vi "Mouse Move (Deprecated).vi"(7 "Map Model in":refnum<class "Map Model.lvclass">, 8 "error in (no error)":errorcluster, 10 "Position":T1, 11 "Eraser in":refnum<class "Eraser.lvclass">) -> (0 "error out":errorcluster, 3 "Eraser out":refnum<class "Eraser.lvclass">, 5 "Map Model out":refnum<class "Map Model.lvclass">)   [LabVIEW 2020, in "Map Model.lvlib" / "Eraser.lvclass"]
uses:
  Eraser.lvclass
  <vilib>/Utility/miscctls.llb/LVPoint32TypeDef.ctl
  Map Model/Map Model.lvclass
  Tool/Tool.lvclass
  Undoable Tool/Undoable Tool.lvclass
  E:/Project/Labview-Projects/Completed projects/Map Editor/Models/Map Model/Tools/Undoable Tool/Undoable Tool.lvclass
  E:/Project/Labview-Projects/Completed projects/Map Editor/Models/Map Model/Tools/Tool/Tool.lvclass
panel:
  # "NOTICE -- YOU MUST LEAVE THIS NOTICE IN PLACE.\n\nCopyright (c) 2017, LIANG LIU Shawn.Liu.cn@gmail.com\nAll rights reserved.\n\nRedistribution and use in source and binary forms, with or without modification, are permitted provided that the following conditions are met:\n-Redistributions of source code must retain the above copyright notice, this list of conditions and the following disclaimer.\n-Redistributions in binary form must reproduce the above copyright notice, this list of conditions and the following disclaimer in the documentation and/or other materials provided with the distribution.\n-Neither the name of the eLp nor the names of its contributors may be used to endorse or promote products derived from this software without specific prior written permission.\n\nTHIS SOFTWARE IS PROVIDED BY THE COPYRIGHT HOLDERS AND CONTRIBUTORS \"AS IS\" AND ANY EXPRESS OR IMPLIED WARRANTIES, INCLUDING, BUT NOT LIMITED TO, THE IMPLIED WARRANTIES OF MERCHANTABILITY AND FITNESS FOR A PARTICULAR PURPOSE ARE DISCLAIMED. IN NO EVENT SHALL THE COPYRIGHT HOLDER OR CONTRIBUTORS BE LIABLE FOR ANY DIRECT, INDIRECT, INCIDENTAL, SPECIAL, EXEMPLARY, OR CONSEQUENTIAL DAMAGES (INCLUDING, BUT NOT LIMITED TO, PROCUREMENT OF SUBSTITUTE GOODS OR SERVICES; LOSS OF USE, DATA, OR PROFITS; OR BUSINESS INTERRUPTION) HOWEVER CAUSED AND ON ANY THEORY OF LIABILITY, WHETHER IN CONTRACT, STRICT LIABILITY, OR TORT (INCLUDING NEGLIGENCE OR OTHERWISE) ARISING IN ANY WAY OUT OF THE USE OF THIS SOFTWARE, EVEN IF ADVISED OF THE POSSIBILITY OF SUCH DAMAGE."
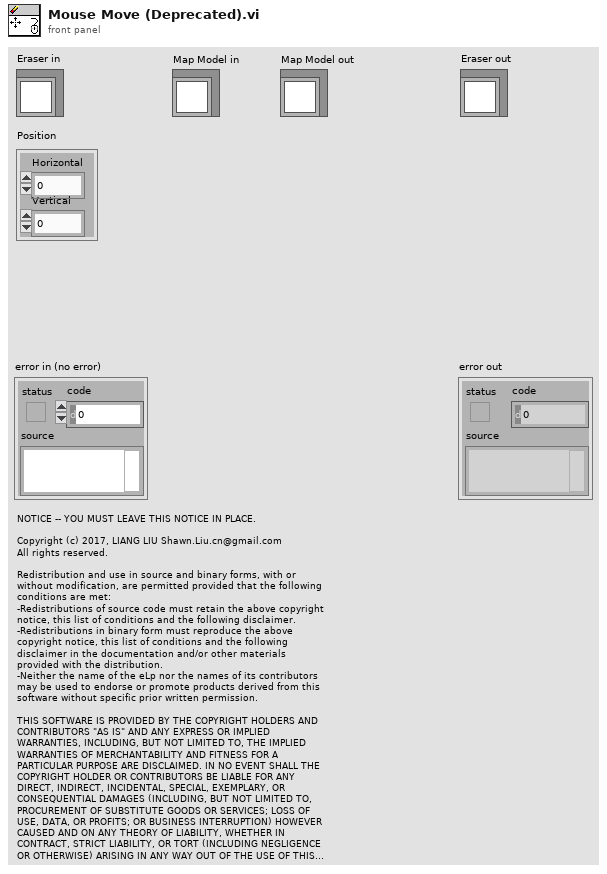
[diagram p1: front panel]
types:
  T1 = typedef "LVPoint32TypeDef.ctl" = cluster{"Horizontal":i32, "Vertical":i32}
  T2 = cluster{"Width":u16, "Style":enum32{"Solid", "Dash", "Dot", "DashDot", "DashDotDot"}}
  T3 = cluster{"Occupied Color":cluster{"Value":u8, "Color":u32}, "Free Color":cluster{"Value":u8, "Color":u32}, "Unknown Color":cluster{"Value":u8, "Color":u32}}
  T4 = typedef "LVPointTypeDef.ctl" = cluster{"Horizontal":i16, "Vertical":i16}
  T5 = typedef "imagedata.ctl" = cluster{"image type":i32, "image depth":i32, "image":u8[], "mask":u8[], "colors":u32[], "Rectangle":cluster{"left":i16, "top":i16, "right":i16, "bottom":i16}}
  T6 = cluster{"left":i16, "top":i16, "right":i16, "bottom":i16}
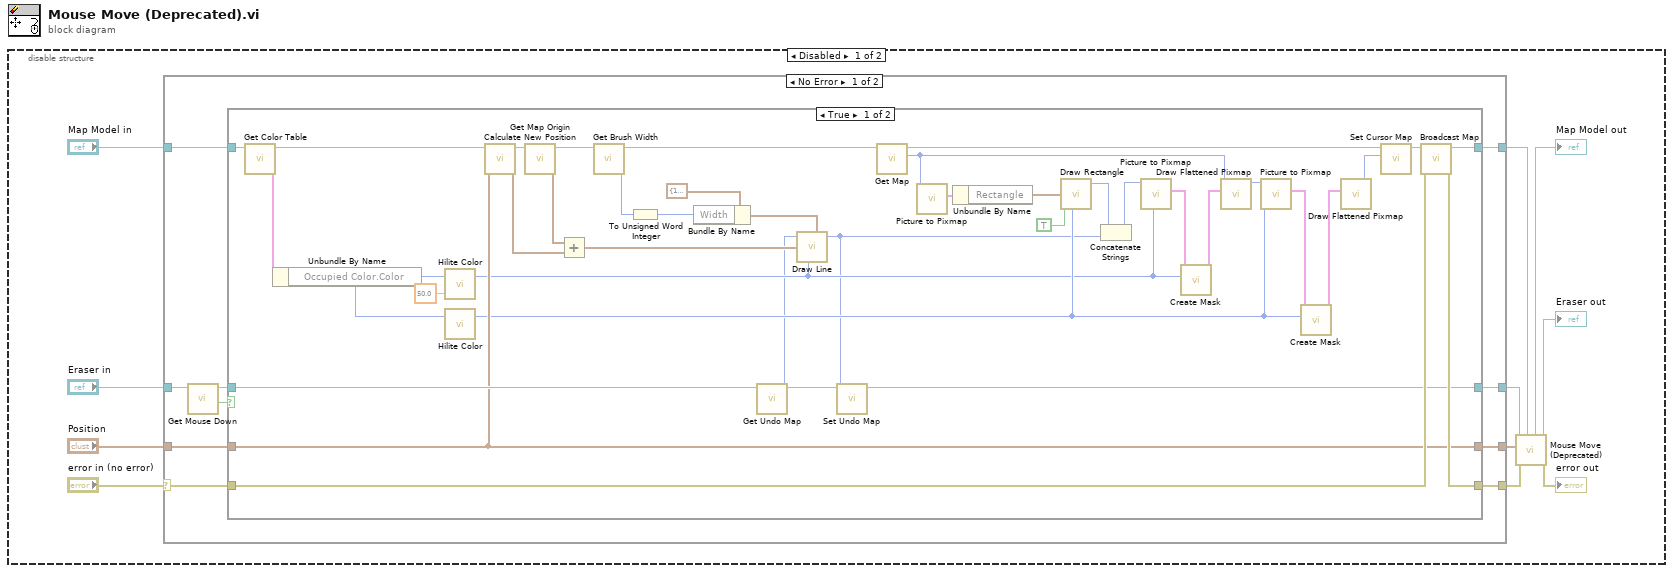
[diagram p0: block diagram]
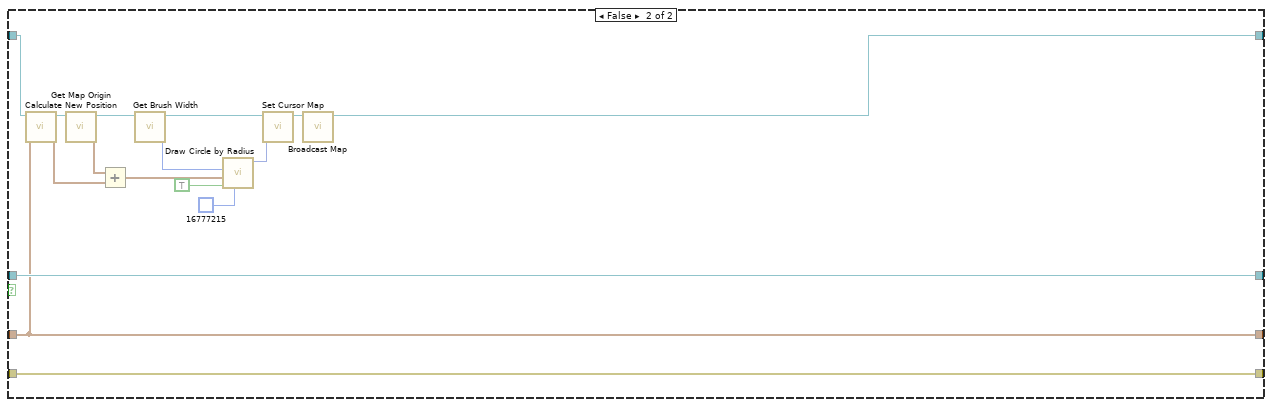
[diagram p2: hidden frame]
diagram:
  n1 = disable-structure shown="Disabled" {
    frame Disabled {
      n2 = case shown="No Error" "error in (no error)" {
        selector: "error in (no error)" -> [w15 w81]
        tunnel: "Map Model in" -> [w21 w80]
        tunnel: [w18 w78] -> w9
        tunnel: [w17 w81] -> w8
        tunnel: "Position" -> [w16 w78]
        tunnel: "Eraser in" -> [w14 w79]
        tunnel: [w13 w80] -> w4
        tunnel: [w12 w79] -> w3
        frame No Error {
          n3 = call "Get Mouse Down.vi"("Tool in"=w14) -> ("Mouse Down"=w19:bool, "Tool out"=w20:refnum<class "Eraser.lvclass">)  [unwired: 9 in]
          n4 = case shown="True" w19 {
            tunnel: w20 -> [w61 w75]
            tunnel: w21 -> [w60 w77]
            tunnel: [w58 w74] -> w13
            tunnel: [w41 w75] -> w12
            tunnel: w16 -> [w44 w63]
            tunnel: [w44 w63] -> w18
            tunnel: w15 -> [w51 w71]
            tunnel: [w50 w71] -> w17
            frame True {
              n5 = call "Get Color Table.vi"("Map Model in"=w60) -> ("Color Table"=w53:T3, "Map Model out"=w54:refnum<class "Map Model.lvclass">)  [unwired: 9 in]
              n6 = Unbundle By Name(w53) -> ("Occupied Color.Color"=w31:u32)
              n7 = call <vilib>:"Hilite Color.vi"("Percentage(30)"=50.0, "Color In"=w31) -> ("Hilite"=w28:u32)  [unwired: 1 out]
              n8 = call <vilib>:"Hilite Color.vi"("Color In"=w31) -> ("Hilite"=w30:u32)  [unwired: 1 in, 1 out]
              n9 = call "Calculate New Position.vi"("Position in"=w44, "Map Model in"=w54) -> ("Position out"=w45:T1, "Map Model out"=w46:refnum<class "Map Model.lvclass">)  [unwired: 8 in]
              n10 = call "Get Map Origin.vi"("Map Model in"=w46) -> ("Map Origin"=w48:T4, "Map Model out"=w49:refnum<class "Map Model.lvclass">)  [unwired: 9 in]
              n11 = Add(x=w48, y=w45) -> (x+y=w43:T1)
              n12 = call "Get Brush Width.vi"("Map Model in"=w49) -> ("Brush Width"=w52:i32, "Map Model out"=w57:refnum<class "Map Model.lvclass">)  [unwired: 9 in]
              n13 = To Unsigned Word Integer(number=w52) -> (unsigned 16bit integer=w27:u16)
              n14 = Bundle By Name(cluster=T2 {"Width"=1, "Style"=enum."Solid"} ("pen"), "Width"=w27) -> (w55:T2)
              n15 = call "Get Undo Map.vi"("Undoable Tool in"=w61) -> ("Undo Map"=w24:picture, "Undoable Tool out"=w42:refnum<class "Eraser.lvclass">)  [unwired: 9 in]
              n16 = call <vilib>:"Draw Line.vi"("picture"=w24, "end point"=w43, "color(black)"=w28, "pen"=w55) -> ("new picture"=w25:picture)  [unwired: 5 in]
              n17 = call "Set Undo Map.vi"("Undo Map"=w25, "Undoable Tool in"=w42) -> ("Undoable Tool out"=w41:refnum<class "Eraser.lvclass">)  [unwired: 9 in]
              n18 = call "Get Map.vi"("Map Model in"=w57) -> ("Map"=w22:picture, "Map Model out"=w40:refnum<class "Map Model.lvclass">)  [unwired: 9 in]
              n19 = call <vilib>:"Picture to Pixmap.vi"("picture"=w22) -> ("image data"=w39:T5)  [unwired: 9 in, 1 out]
              n20 = Unbundle By Name(w39) -> ("Rectangle"=w38:T6)
              n21 = call <vilib>:"Draw Rectangle.vi"("rect"=w38, "fill?(F)"=TRUE, "color(black)"=w30) -> ("new picture"=w37:picture)  [unwired: 6 in]
              n22 = Concatenate Strings(w37, w25) -> (w29:picture)
              n23 = call <vilib>:"Picture to Pixmap.vi"("Background Color"=w28, "picture"=w29) -> ("image data"=w36:T5)  [unwired: 8 in, 1 out]
              n24 = call <vilib>:"Create Mask.vi"("Mask Color (Black)"=w28, "image data"=w36) -> ("image data"=w35:T5)  [unwired: 9 in]
              n25 = call <vilib>:"Draw Flattened Pixmap.vi"("image data"=w35, "picture"=w22) -> ("new picture"=w32:picture)  [unwired: 7 in]
              n26 = call <vilib>:"Picture to Pixmap.vi"("Background Color"=w30, "picture"=w32) -> ("image data"=w33:T5)  [unwired: 8 in, 1 out]
              n27 = call <vilib>:"Create Mask.vi"("Mask Color (Black)"=w30, "image data"=w33) -> ("image data"=w34:T5)  [unwired: 9 in]
              n28 = call <vilib>:"Draw Flattened Pixmap.vi"("image data"=w34) -> ("new picture"=w23:picture)  [unwired: 8 in]
              n29 = call "Set Cursor Map.vi"("Cursor Map"=w23, "Map Model in"=w40) -> ("Map Model out"=w59:refnum<class "Map Model.lvclass">)  [unwired: 9 in]
              n30 = call "Broadcast Map.vi"("error in (no error)"=w51, "Map Model in"=w59) -> ("error out"=w50:errorcluster, "Map Model out"=w58:refnum<class "Map Model.lvclass">)  [unwired: 8 in]
            }
            frame False {
              n31 = call "Calculate New Position.vi"("Position in"=w63, "Map Model in"=w77) -> ("Position out"=w62:T1, "Map Model out"=w64:refnum<class "Map Model.lvclass">)  [unwired: 8 in]
              n32 = call "Get Map Origin.vi"("Map Model in"=w64) -> ("Map Origin"=w66:T4, "Map Model out"=w67:refnum<class "Map Model.lvclass">)  [unwired: 9 in]
              n33 = Add(x=w66, y=w62) -> (x+y=w65:T1)
              n34 = call "Get Brush Width.vi"("Map Model in"=w67) -> ("Brush Width"=w69:i32, "Map Model out"=w70:refnum<class "Map Model.lvclass">)  [unwired: 9 in]
              n35 = call <vilib>:"Draw Circle by Radius.vi"("color(black)"=u32 16777215, "fill?(F)"=TRUE, "pixel center"=w65, "radius"=w69) -> ("new picture"=w73:picture)  [unwired: 7 in]
              n36 = call "Set Cursor Map.vi"("Cursor Map"=w73, "Map Model in"=w70) -> ("Map Model out"=w76:refnum<class "Map Model.lvclass">)  [unwired: 9 in]
              n37 = call "Broadcast Map.vi"("Map Model in"=w76) -> ("Map Model out"=w74:refnum<class "Map Model.lvclass">)  [unwired: 9 in, 1 out]
            }
          }
        }
        frame Error {
        }
      }
      n38 = call-parent "Mouse Move (Deprecated).vi"("Map Model in"=w4, "error in (no error)"=w8, "Position"=w9, "Tool in"=w3) -> ("error out"=→"error out":errorcluster, "Tool out"=→"Eraser out":refnum<class "Eraser.lvclass">, "Map Model out"=→"Map Model out":refnum<class "Map Model.lvclass">)  [unwired: 5 in]
    }
    frame Enabled {
    }
  }
